vi "CoboltLaser_LaserOnOffStateGet.vi"(0 "ComPort":refnum<visa-resource-name>, 3 "GenerateError":bool=TRUE, 7 "error in (no error)":errorcluster) -> (20 "ComPortOut":refnum<visa-resource-name>, 21 "On":bool, 22 "Response":string, 23 "ResponseOK":bool, 27 "error out":errorcluster)   [LabVIEW 2019]
doc: "Use this template to build a VI to use as a subVI."
uses:
  <userlib>/CoboltLaser/CoboltLaser_Controls/ExpectedResponseType.ctl
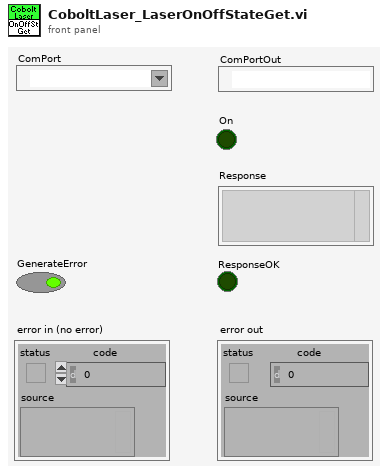
[diagram p1: front panel]
types:
  T1 = typedef "ExpectedResponseType.ctl" = enum16{"Any", "Digits Only", "Non-Digits Only"}
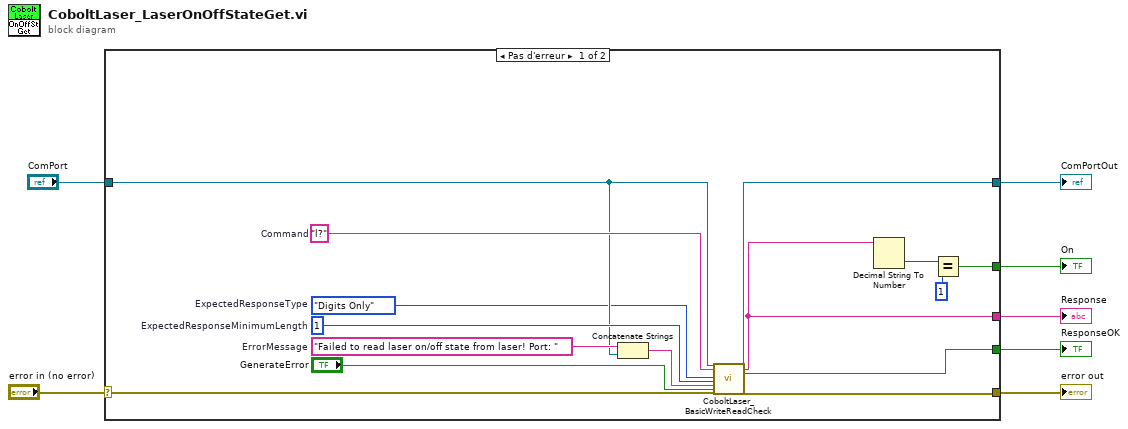
[diagram p0: block diagram]
diagram:
  n1 = case shown="Pas d'erreur" "error in (no error)" {
    selector: "error in (no error)" -> [w22 w24]
    tunnel: [w21 w24] -> w6
    tunnel: "ComPort" -> [w13 w23]
    tunnel: [w12 w23] -> w4
    tunnel: [w11 _] -> w3
    tunnel: [w10 _] -> w2
    tunnel: [w9 _] -> w1
    frame No Error {
      w8 = ExpectedResponseType."Digits Only"  # ExpectedResponseType
      w19 = 1  # ExpectedResponseMinimumLength
      w17 = "Failed to read laser on/off state from laser! Port: "  # ErrorMessage
      w20 = "l?"  # Command
      n2 = Concatenate Strings(w17, w13) -> (w16:string)
      n3 = call <userlib>:"CoboltLaser_BasicWriteReadCheck.vi"("ComPort"=w13, "Command"=w20, "ExpectedResponseType"=w8, "ExpectedResponseMinimumLength"=w19, "ErrorMessage"=w16, "GenerateError"="GenerateError", "error in (no error)"=w22) -> ("ComPortOut"=w12:refnum<visa-resource-name>, "Response"=w10:string, "ResponseOK"=w9:bool, "error out"=w21:errorcluster)  [unwired: 17 in]
      n4 = Decimal String To Number(string=w10) -> (number=w15:i32)  [unwired: 2 in, 1 out]
      n5 = Equal?(x=w15, y=1) -> (x = y?=w11:bool)
    }
    frame Error {
    }
  }
  "error out" <- w6
  "ComPortOut" <- w4
  "Response" <- w2
  "ResponseOK" <- w1
  "On" <- w3
